vi "APC_9056_additonalSignals.vi"() -> (0 "AdditionalTSSignalList_post":string[](array[string])=["NI9264_AO0_V", "NI9264_AO1_V", "NI9264_AO2_V", "NI9264_AO3_V", "NI9264_AO4_V", "NI9264_AO5_V", "NI9264_AO6_V", "NI9264_AO7_V", "NI9264_AO8_V", "NI9264_AO9_V", "NI9264_AO10_V", "NI9264_AO11_V", "NI9264_AO12_V", "NI9264_AO13_V", "NI9264_AO14_V", "NI9264_AO15_V", "O2-FC-001-REF_mA", "AR-PC-002-REF_mA", "NG-FC-001-REF_mA", "EC-FC-001_mA", "SW-FC-004-REF_mA", "SW-FC-009_mA", "DYNO-REF_mA", "NI9266_AO7_mA", "NG-FV-001_b", "O2-PV-004_b", "AR-PV-004_b", "WF-FC-001_b", "WF-FC-002_b", "WF-FC-003_b", "NI9375_AO6_b", "NI9375_AO7_b", "NI9375_AO8_b", "NI9375_AO9_b", "NI9375_AO10_b", "NI9375_AO11_b", "NI9375_AO12_b", "NI9375_AO13_b", "NI9375_AO14_b", "NI9375_AO15_b", "NI9375_AI0_b", "NI9375_AI1_b", "NI9375_AI2_b", "NI9375_AI3_b", "NI9375_AI4_b", "NI9375_AI5_b", "NI9375_AI6_b", "NI9375_AI7_b", "NI9375_AI8_b", "NI9375_AI9_b", "NI9375_AI10_b", "NI9375_AI11_b", "NI9375_AI12_b", "NI9375_AI13_b", "NI9375_AI14_b", "NI9375_AI15_b"], 1 "AdditionalTSSignalList_pre":string[](array[string])=["TimeStamp9056_ms", "SystemState_i8"])   [LabVIEW 2020]
panel:
  in  "From PC":string[](array[string])=["AIC103_CO2_ConcTarget_ack", "AT103_CO2Conc", "PV103_PressTarget_kPa_ack", "PT103_Pressure_kPa", "PV103_VlvPosTarget_pc_ack", "PV103_VlvPos_pc_fb", "AIC201_CO2_ConcTarget_ack", "AT201_CO2Conc", "FV301_FlowTarget_kgh_ack", "FT301_Flow_kgh", "FV301_VlvPosTarget_pc_ack", "FV301_VlvPos_pc_fb", "PV300_PressTarget_kPa_ack", "PT300_Pressure_kPa", "PV300_VlvPosTarget_pc_ack", "PV300_VlvPos_pc_fb", "C101_CompSpeed_rpm", "PT104_Pressure_kPa", "PT106_Pressure_kPa", "PLC_Manual_Control", "MTR_State", "MTR_HeartBeat", "PV103_Ctrl_Mode_act", "FV301_Ctrl_Mode_act", "PV300_Ctrl_Mode_act", "MTR_Diagnostic_Status"]
  in  "NI9375_DI":string[](array[string])=["NI9375_AI0_b", "NI9375_AI1_b", "NI9375_AI2_b", "NI9375_AI3_b", "NI9375_AI4_b", "NI9375_AI5_b", "NI9375_AI6_b", "NI9375_AI7_b", "NI9375_AI8_b", "NI9375_AI9_b", "NI9375_AI10_b", "NI9375_AI11_b", "NI9375_AI12_b", "NI9375_AI13_b", "NI9375_AI14_b", "NI9375_AI15_b"]
  in  "NI9266":string[](array[string])=["O2-FC-001-REF_mA", "AR-PC-002-REF_mA", "NG-FC-001-REF_mA", "EC-FC-001_mA", "SW-FC-004-REF_mA", "SW-FC-009_mA", "DYNO-REF_mA", "NI9266_AO7_mA"]
  in  "NI9375_DO":string[](array[string])=["NG-FV-001_b", "O2-PV-004_b", "AR-PV-004_b", "WF-FC-001_b", "WF-FC-002_b", "WF-FC-003_b", "NI9375_AO6_b", "NI9375_AO7_b", "NI9375_AO8_b", "NI9375_AO9_b", "NI9375_AO10_b", "NI9375_AO11_b", "NI9375_AO12_b", "NI9375_AO13_b", "NI9375_AO14_b", "NI9375_AO15_b"]
  in  "NI9264":string[](array[string])=["NI9264_AO0_V", "NI9264_AO1_V", "NI9264_AO2_V", "NI9264_AO3_V", "NI9264_AO4_V", "NI9264_AO5_V", "NI9264_AO6_V", "NI9264_AO7_V", "NI9264_AO8_V", "NI9264_AO9_V", "NI9264_AO10_V", "NI9264_AO11_V", "NI9264_AO12_V", "NI9264_AO13_V", "NI9264_AO14_V", "NI9264_AO15_V"]
  in  "Signal raster previous to the AI":string[](array[string])=["TimeStamp9056_ms", "SystemState_i8"]
  # "NAMING: for calculated and OUTPUT variables , include units on variable names.\n\n_bar \n_degC      (ºC)\n_perc       (%)\n_rpm\n_r              (ratio)\n_b             (bool)\n_u64"
  # "NI9056"
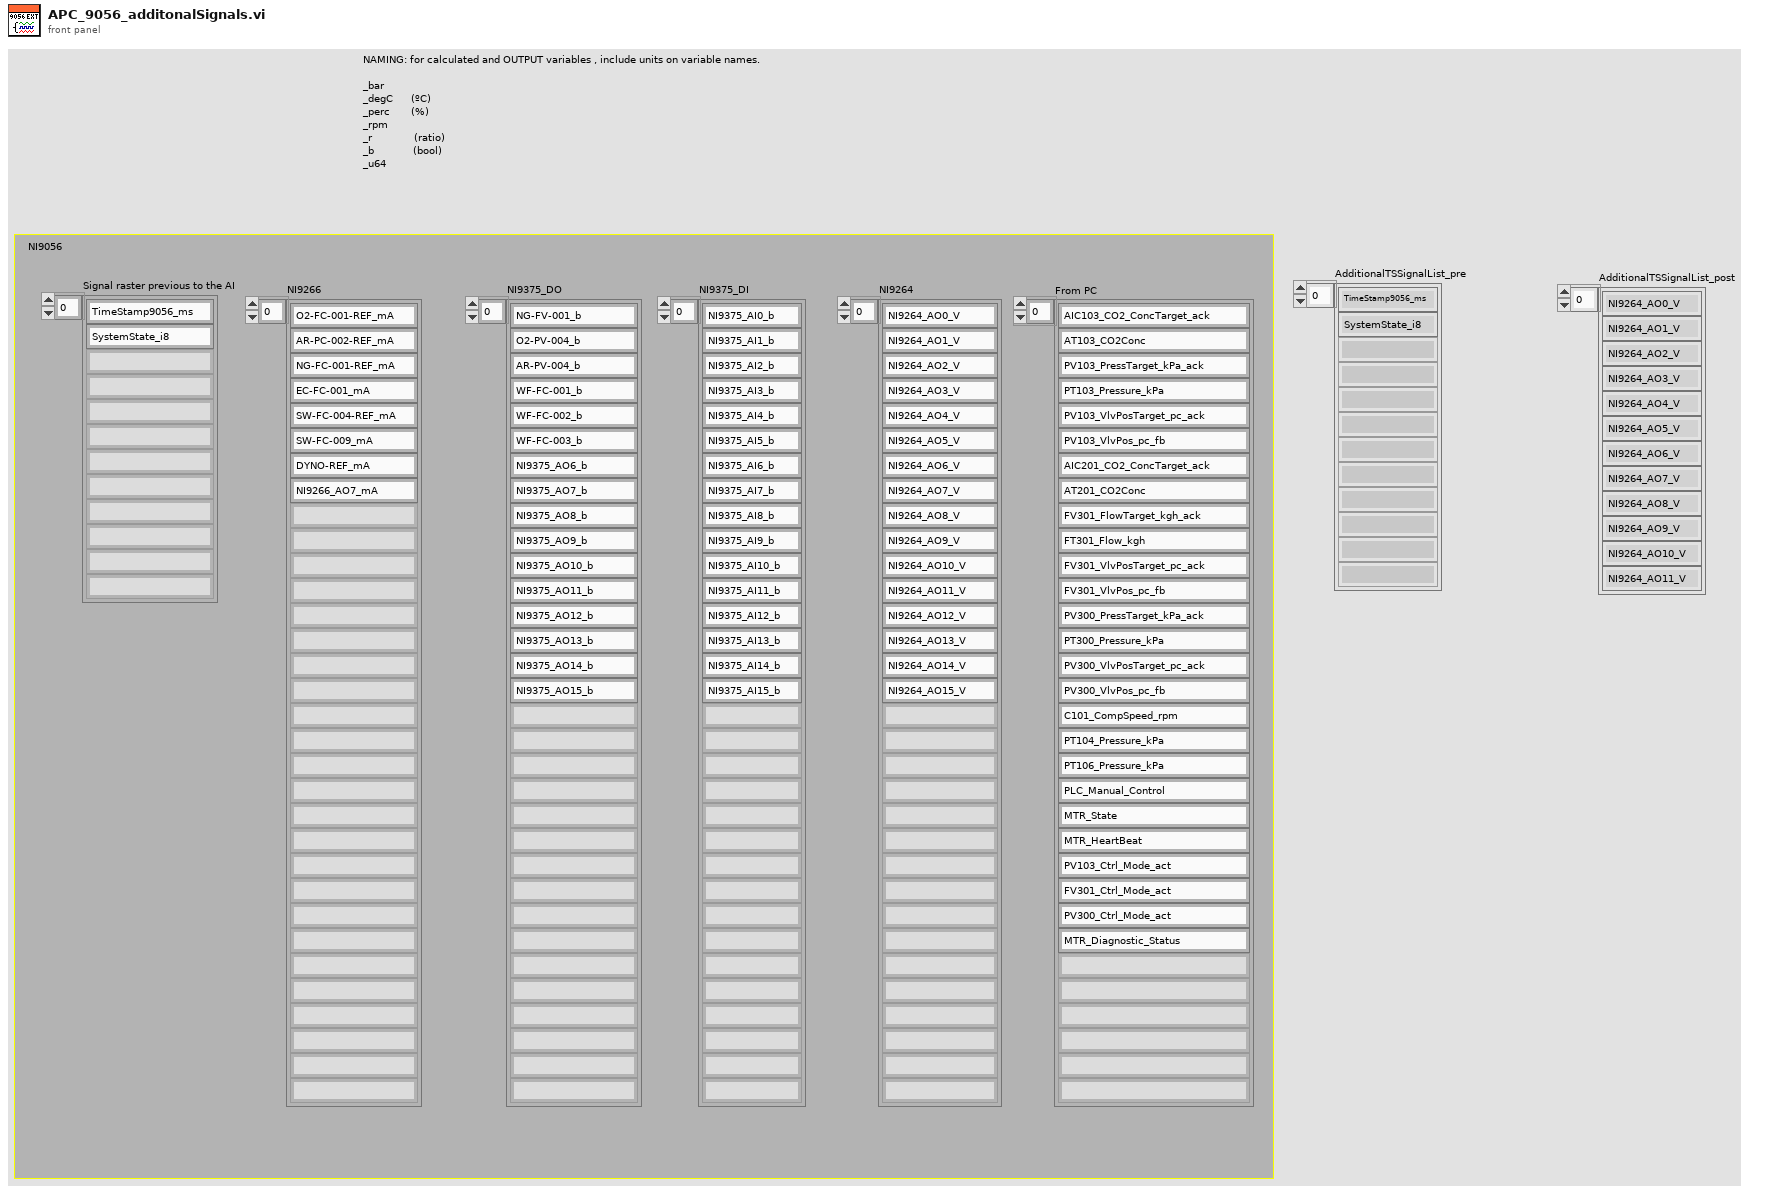
[diagram p1: front panel]
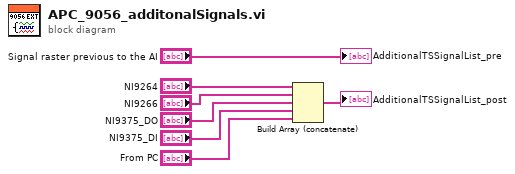
[diagram p0: block diagram]
diagram:
  n1 = Build Array (concatenate)("NI9264", "NI9266", "NI9375_DO", "NI9375_DI", "From PC") -> (→"AdditionalTSSignalList_post":string[])
  "AdditionalTSSignalList_pre" <- "Signal raster previous to the AI"
